vi "Button Definition JSON File Parse Error.vi"(11 "Button Def JSON":path) -> (0 "error out":errorcluster)   [LabVIEW 2020, in "Navigation.lvlib" / "Button Manager.lvclass"]
doc: "____\nHAMPEL SOFTWARE ENGINEERING v2.6.0 (2023-12-19 10:54)"
uses:
  Button Manager.lvclass
  Button Manager.lvclass/Button Manager.ctl
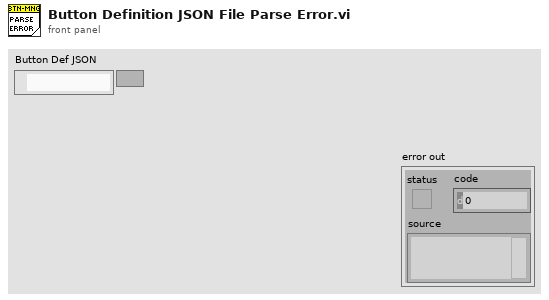
[diagram p1: front panel]
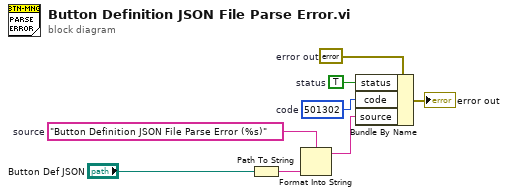
[diagram p0: block diagram]
diagram:
  w5 = errorcluster {"status"=FALSE, "code"=0, "source"=""}  # error out
  w1 = TRUE  # status
  w3 = 501302  # code
  w8 = "Button Definition JSON File Parse Error (%s)"  # source
  n1 = Path To String(path="Button Def JSON") -> (string=w6:string)
  n2 = Format Into String(format string=w8, w6) -> (resulting string=w2:string)  [unwired: 2 in, 1 out]
  n3 = Bundle By Name(cluster=w5, "status"=w1, "code"=w3, "source"=w2) -> (→"error out":errorcluster)
